vi "u64.be.vi"(8 "end":u8=14, 9 "start":u8=6, 10 "Data":u8, 11 "Counter":u8) -> (3 "Latched\nValue":u64)   [LabVIEW 2022 SP3]
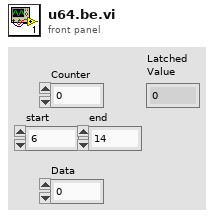
[diagram p1: front panel]
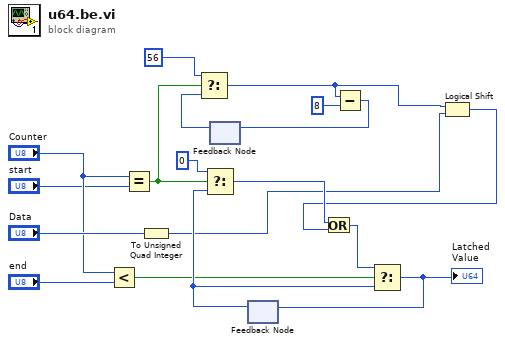
[diagram p0: block diagram]
diagram:
  n1 = Less?(x="Counter", y="end") -> (x < y?=w12:bool)
  n2 = Equal?(x="Counter", y="start") -> (x = y?=w8:bool)
  n3 = To Unsigned Quad Integer(1:"Data") -> (0:w2:u64)
  n4 = feedback #1() -> (w6:i16)  [unwired: 1 in]
  n5 = Select(t=i16 56 ("y"), s=w8, f=w6) -> (s? t:f=w3:i16)
  n6 = feedback #2() -> (w14:u64)  [unwired: 1 in]
  n7 = Select(t=u64 0 ("y"), s=w8, f=w14) -> (s? t:f=w16:u64)
  n8 = Subtract(x=w3, y=i16 8) -> (x-y=w4:i16)
  n9 = feedback-in #1(w4) -> ()
  n10 = Logical Shift(y=w3, x=w2) -> (x << y=w1:u64)
  n11 = Or(x=w16, y=w1) -> (x .or. y?=w17:u64)
  n12 = Select(t=w17, s=w12, f=w14) -> (s? t:f=w18:u64)
  "Latched\nValue" <- w18
  n13 = feedback-in #2(w18) -> ()
